vi "decision.vi"(8 "offset":dbl, 10 "weights":dbl[](array[numeric]), 11 "inputs":dbl[](array[numeric])) -> (2 "decision":dbl)   [LabVIEW 2014]
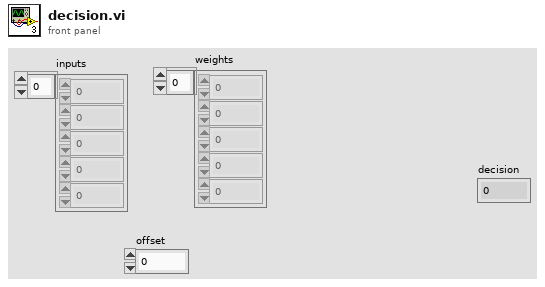
[diagram p1: front panel]
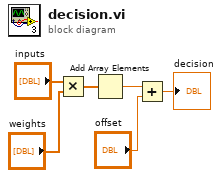
[diagram p0: block diagram]
diagram:
  n1 = Multiply(x="inputs", y="weights") -> (x*y=w4:dbl[])
  n2 = Add Array Elements(numeric array=w4) -> (sum=w3:dbl)
  n3 = Add(x=w3, y="offset") -> (x+y=→"decision":dbl)
